vi "Get path (relative-base).vi"(6 "Strip lead \"/\" (F)":bool, 8 "error in (no error)":errorcluster, 9 "Encoded? (F)":bool, 11 "URI-Component.Path in":refnum<class "URI-Component.Path.lvclass">) -> (0 "error out":errorcluster, 1 "common-path":string, 2 "relative-path":string, 3 "URI-Component.Path out":refnum<class "URI-Component.Path.lvclass">)   [LabVIEW 2013, in "openURI.lvlib" / "URI-Component.Path.lvclass"]
uses:
  URI-Component.Path.lvclass
  URI-Component.Path.lvclass/URI-Component.Path.ctl
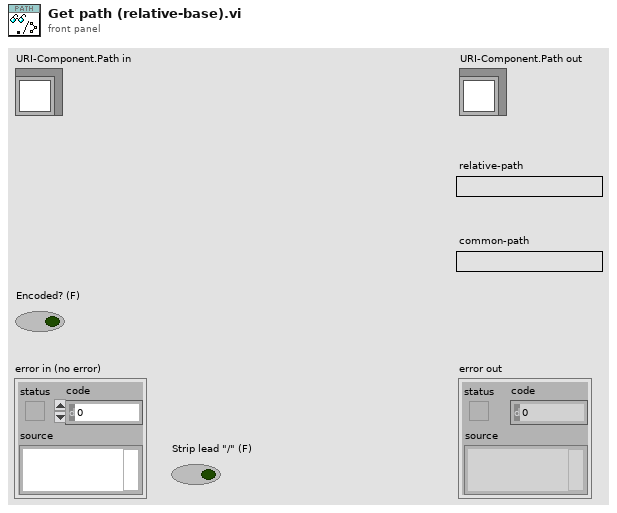
[diagram p1: front panel]
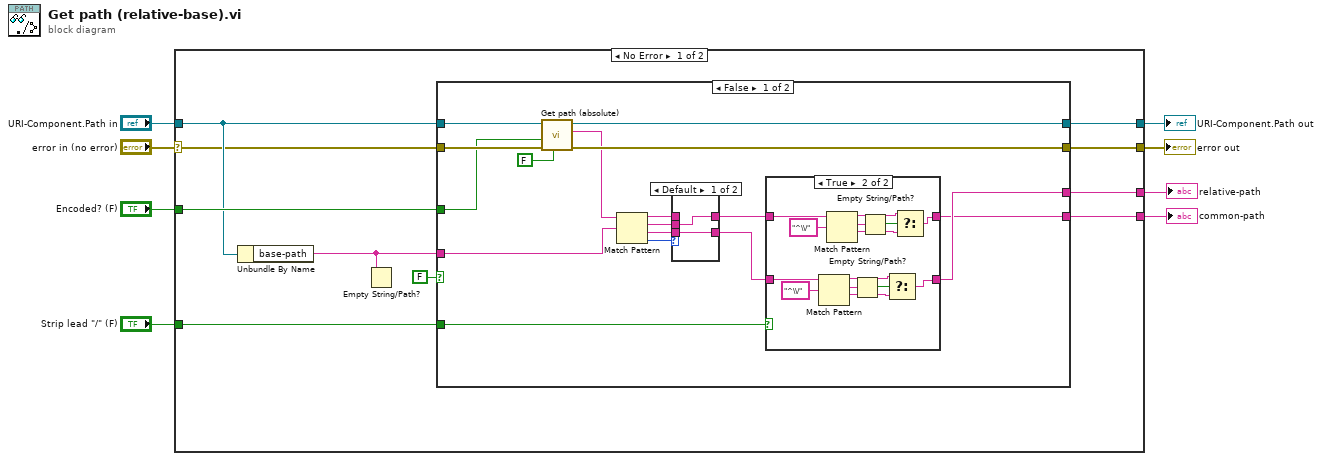
[diagram p0: block diagram]
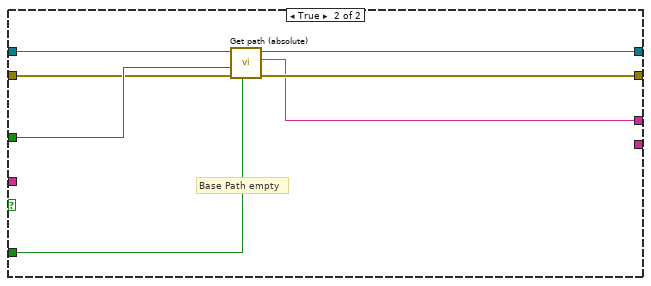
[diagram p4: hidden frame]
diagram:
  n1 = case shown="No Error" "error in (no error)" {
    selector: "error in (no error)" -> [w15 w63]
    tunnel: [w14 w63] -> w7
    tunnel: [w13 w62] -> w5
    tunnel: "URI-Component.Path in" -> [w16 w62]
    tunnel: [w12 _] -> w4
    tunnel: "Encoded? (F)" -> [w18 _]
    tunnel: "Strip lead \"/\" (F)" -> [w17 _]
    tunnel: [w11 _] -> w1
    frame No Error {
      n2 = Unbundle By Name(w16) -> ("base-path"=w10:string)
      n3 = Empty String/Path?(string/path=w10) -> ()  [unwired: 1 out]
      n4 = case shown="False" FALSE {
        tunnel: w10 -> [w20 _]
        tunnel: w16 -> [w35 w61]
        tunnel: w18 -> [w33 w60]
        tunnel: w17 -> [w23 w59]
        tunnel: w15 -> [w34 w58]
        tunnel: [w30 w57] -> w14
        tunnel: [w31 w56] -> w13
        tunnel: [w24 w55] -> w12
        tunnel: [w21 _] -> w11
        frame False {
          n5 = call "Get path (absolute).vi"("Strip lead \"/\" (F)"=FALSE ("Strip lead \"/\" (F)"), "error in (no error)"=w34, "Encoded? (F)"=w33, "URI-Component.Path in"=w35) -> ("error out"=w30:errorcluster, "path-component"=w19:string, "URI-Component.Path out"=w31:refnum<class "URI-Component.Path.lvclass">)  [unwired: 5 in]
          n6 = Match Pattern(string=w19, regular expression=w20) -> (before substring=w28:string, match substring=w26:string, after substring=w27:string, offset past match=w29:i32)  [unwired: 1 in]
          n7 = case shown="Default" w29 {
            tunnel: [w52 _] -> w22
            tunnel: w28 -> [_ w54]
            tunnel: [w53 w54] -> w25
            tunnel: w27 -> [w53 _]
            tunnel: w26 -> [w52 _]
            frame Default {
            }
            frame -1 {
            }
          }
          n8 = case shown="True" w23 {
            tunnel: w25 -> [w36 w50]
            tunnel: [w36 w45] -> w24
            tunnel: w22 -> [w37 w39]
            tunnel: [w37 w38] -> w21
            frame False {
            }
            frame True {
              n9 = Match Pattern(string=w50, regular expression="^\\/") -> (before substring=w47:string, match substring=w49:string, after substring=w46:string)  [unwired: 1 in, 1 out]
              n10 = Match Pattern(string=w39, regular expression="^\\/") -> (before substring=w43:string, match substring=w41:string, after substring=w44:string)  [unwired: 1 in, 1 out]
              n11 = Empty String/Path?(string/path=w49) -> (empty?=w48:bool)
              n12 = Empty String/Path?(string/path=w41) -> (empty?=w42:bool)
              n13 = Select(t=w47, s=w48, f=w46) -> (s? t:f=w45:string)
              n14 = Select(t=w43, s=w42, f=w44) -> (s? t:f=w38:string)
            }
          }
        }
        frame True {
          # "Base Path empty"
          n15 = call "Get path (absolute).vi"("Strip lead \"/\" (F)"=w59, "error in (no error)"=w58, "Encoded? (F)"=w60, "URI-Component.Path in"=w61) -> ("error out"=w57:errorcluster, "path-component"=w55:string, "URI-Component.Path out"=w56:refnum<class "URI-Component.Path.lvclass">)  [unwired: 5 in]
        }
      }
    }
    frame Error {
    }
  }
  "error out" <- w7
  "URI-Component.Path out" <- w5
  "relative-path" <- w4
  "common-path" <- w1
